vi "CheckValidReportPath.vi"(8 "Error In":errorcluster, 11 "AutoData":T1) -> (0 "Error Out":errorcluster, 3 "AutoData out":T1)   [LabVIEW 2019, in "AutoMode.lvlib"]
uses:
  AutoMode.lvlib
  Cluster - AutoModeData.ctl
  MainController/Cluster - TestSettings.ctl
  MainController/Cluster - HardwareConfiguration.ctl
  MainController/Cluster - TestResults.ctl
  Cluster - AutoModeMessage.ctl
  Enum - AutoModeState.ctl
  MainController/Cluster - MainControllerMessage.ctl
  MainController/Enum - MainState.ctl
  EventLogger/EventLogger.lvlib
  MainController/MainController.lvlib
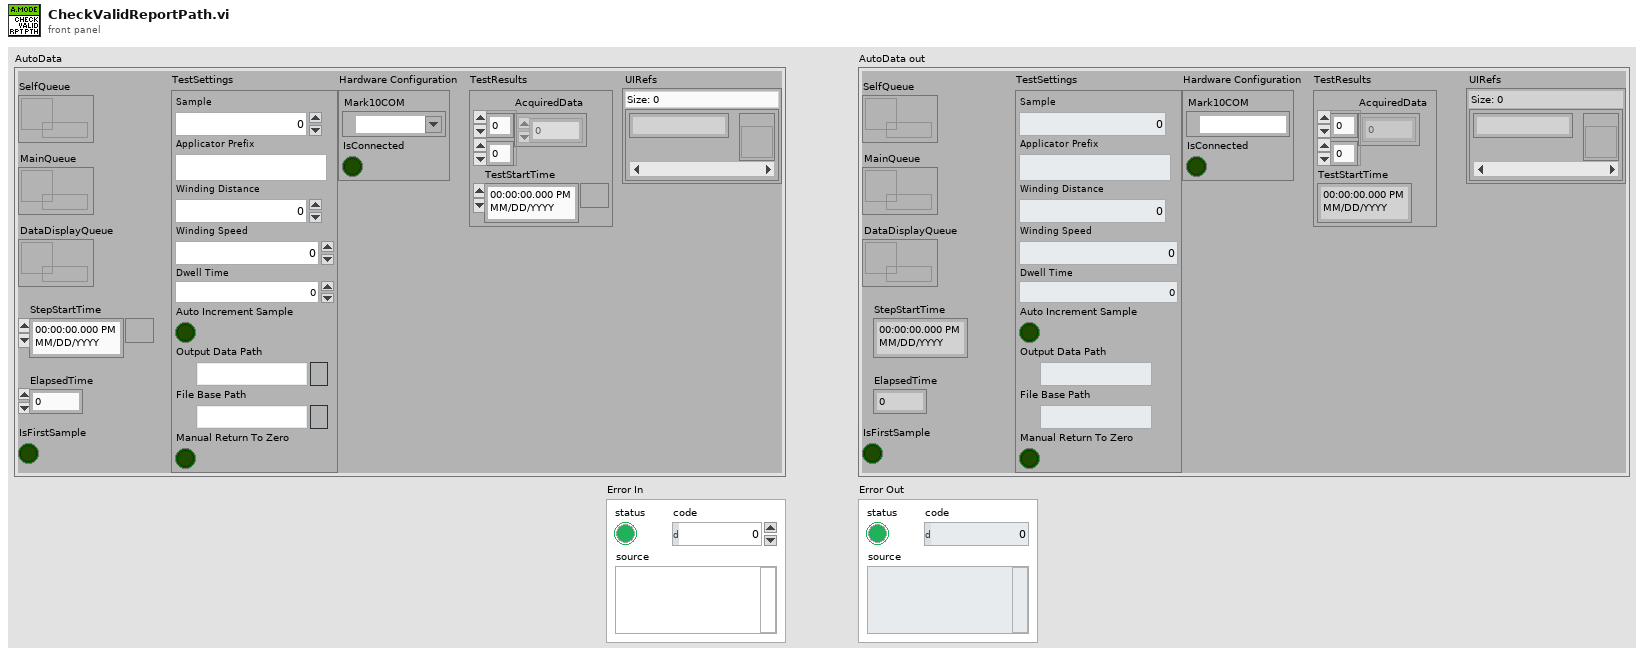
[diagram p1: front panel]
types:
  T1 = typedef "AutoMode.lvlib/Cluster - AutoModeData.ctl" = cluster{"DataDisplayQueue":refnum<queue>, "StepStartTime":timestamp, "TestSettings":T2, "Hardware Configuration":T3, "TestResults":T4, "ElapsedTime":dbl, "IsFirstSample":bool, "SelfQueue":refnum<queue>, "MainQueue":refnum<queue>, "UIRefs":map{string, refnum<vi>}}
  T2 = typedef "MainController.lvlib/Cluster - TestSettings.ctl" = cluster{"Sample":u32, "Applicator Prefix":string, "Winding Distance":dbl, "Winding Speed":dbl, "Dwell Time":dbl, "Auto Increment Sample":bool, "Output Data Path":path, "File Base Path":path, "Manual Return To Zero":bool}
  T3 = typedef "MainController.lvlib/Cluster - HardwareConfiguration.ctl" = cluster{"Mark10COM":refnum<visa-resource-name>, "IsConnected":bool}
  T4 = typedef "MainController.lvlib/Cluster - TestResults.ctl" = cluster{"AcquiredData":dbl[][], "TestStartTime":timestamp}
  T5 = typedef "AutoMode.lvlib/Enum - AutoModeState.ctl" = enum16{"Initialize", "Idle", "UpdateConfig", "UpdateHWConfig", "BroadcastSettings", "Start", "CheckValidReportPath", "Winding", "WaitForWinding", "Unwind", "WaitForUnwind", "Stop", "Abort", "WriteDataToFile", "EventTriggered", "GenerateFilePath", "ZeroPosition", "GotoZero", "Error", "Exit"}
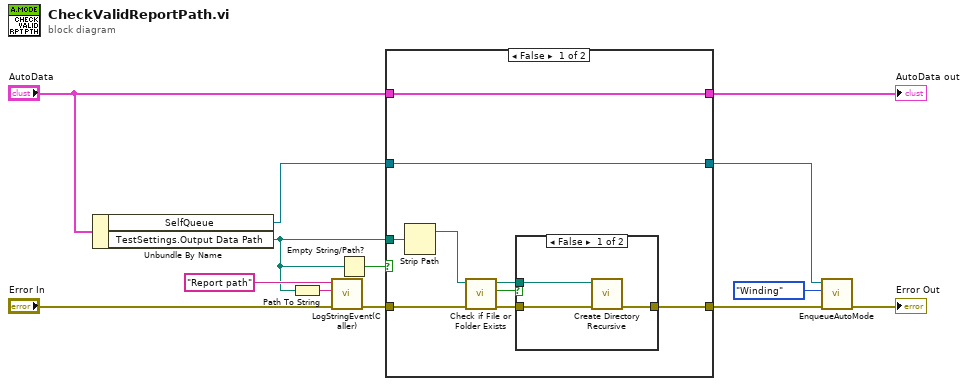
[diagram p0: block diagram]
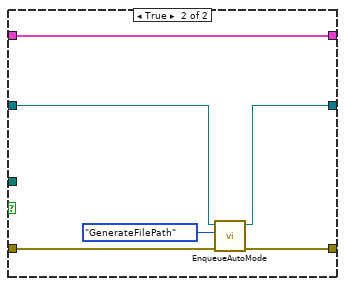
[diagram p3: hidden frame]
diagram:
  n1 = Unbundle By Name("AutoData") -> ("SelfQueue"=w7:refnum<queue>, "TestSettings.Output Data Path"=w2:path)
  n2 = Path To String(path=w2) -> (string=w1:string)
  n3 = call "LogStringEvent(Caller).vi"("Error In"="Error In", "Data"=w1, "Field"="Report path") -> ("Error Out"=w4:errorcluster)  [unwired: 8 in]
  n4 = Empty String/Path?(string/path=w2) -> (empty?=w9:bool)
  n5 = case shown="False" w9 {
    tunnel: [w21 w30] -> w13
    tunnel: w4 -> [w17 w31]
    tunnel: w2 -> [w16 _]
    tunnel: [w15 w29] -> w8
    tunnel: w7 -> [w15 w28]
    tunnel: "AutoData" -> [w14 w27]
    tunnel: [w14 w27] -> w5
    frame False {
      n6 = Strip Path(path=w16) -> (stripped path=w22:path)  [unwired: 1 out]
      n7 = call <vilib>:"Check if File or Folder Exists.vi"("error in (no error)"=w17, "path"=w22) -> ("error out"=w20:errorcluster, "file or folder exists?"=w19:bool, "dup path"=w18:path)  [unwired: 7 in]
      n8 = case shown="False" w19 {
        tunnel: [w24 w26] -> w21
        tunnel: w20 -> [w25 w26]
        tunnel: w18 -> [w23 _]
        frame False {
          n9 = call <vilib>:"Create Directory Recursive.vi"("error in (no error)"=w25, "directory"=w23) -> ("error out"=w24:errorcluster)  [unwired: 3 in, 2 out]
        }
        frame True {
        }
      }
    }
    frame True {
      n10 = call "EnqueueAutoMode.vi"("error in (no error)"=w31, "AutoState"=Enum_-_AutoModeState."GenerateFilePath", "Queue in"=w28) -> ("error out"=w30:errorcluster, "queue out"=w29:refnum<queue>)  [unwired: 7 in]
    }
  }
  "AutoData out" <- w5
  n11 = call "EnqueueAutoMode.vi"("error in (no error)"=w13, "AutoState"=Enum_-_AutoModeState."Winding", "Queue in"=w8) -> ("error out"=→"Error Out":errorcluster)  [unwired: 7 in, 1 out]
